vi "Configure Dialog.vi"(8 "error in (no error)":errorcluster, 11 "CAN Port Configuration in":T1={"CAN Interface"="CAN1", "XNET Cluster"="NIXNET_example.CAN_Cluster", "#Signals"=0, "Sample Rate (Hz)"=100.0} {"Sample Rate (Hz)" format="%#_13g"}) -> (0 "error out":errorcluster, 1 "Canceled?":bool, 3 "CAN Port Configuration out":T1={"CAN Interface"="CAN1", "XNET Cluster"="NIXNET_example.CAN_Cluster", "#Signals"=28, "Sample Rate (Hz)"=100.0} {"Sample Rate (Hz)" format="%#_13g"})   [LabVIEW 2021, in "XNET-CAN-Signal-Logger.lvlib"]
uses:
  XNET-CAN-Signal-Logger.lvlib
  Typedef/Def-CAN Port Configuration.ctl
  <resource>/objmgr/xnet.rc
panel:
  in  "Cancel":bool
  in  "OK":bool
  in  "CAN Port Configuration":T1={"CAN Interface"="CAN1", "XNET Cluster"="ManyXnetChannels", "#Signals"=0, "Sample Rate (Hz)"=100.0} {"Sample Rate (Hz)" format="%#_13g"}
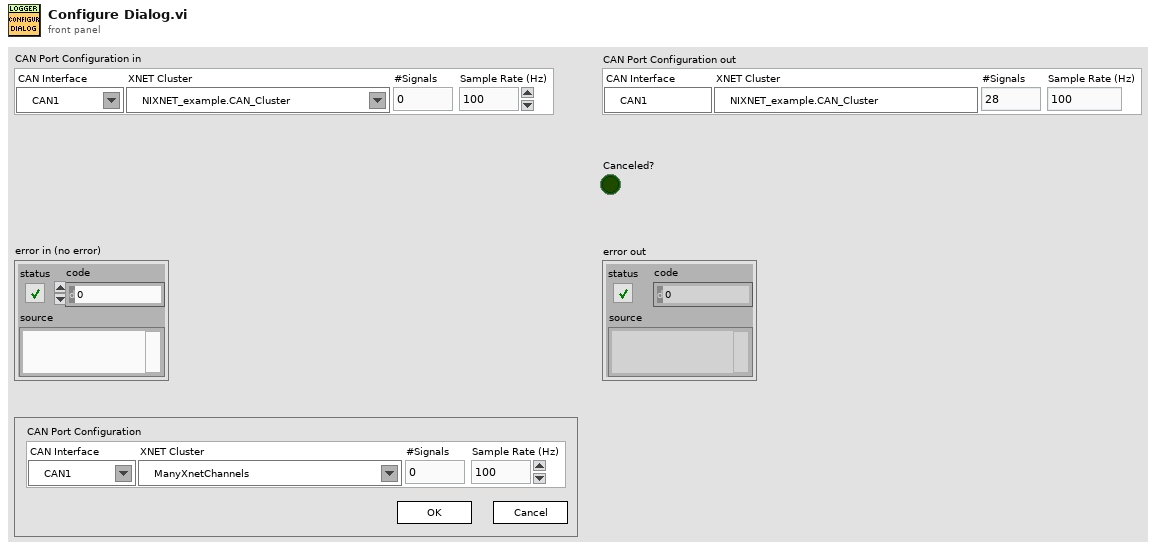
[diagram p1: front panel]
types:
  T1 = typedef "XNET-CAN-Signal-Logger.lvlib/Def-CAN Port Configuration.ctl" = cluster{"CAN Interface":refnum<k21>, "XNET Cluster":refnum<k21>, "#Signals":i32, "Sample Rate (Hz)":dbl}
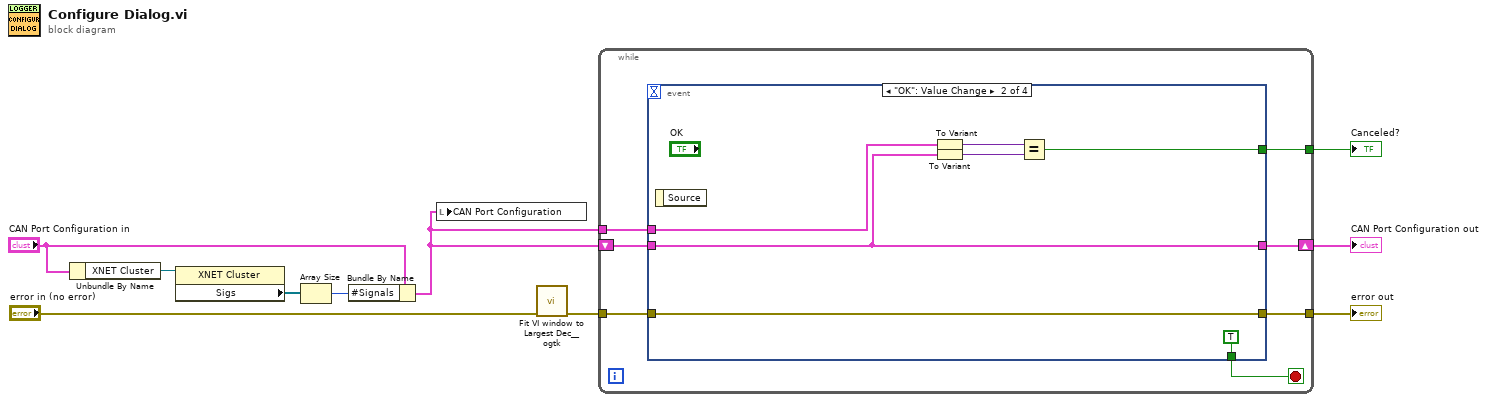
[diagram p0: block diagram]
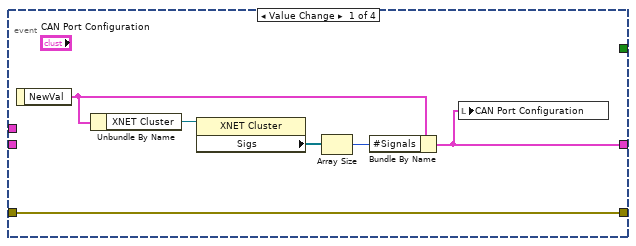
[diagram p2: hidden frame]
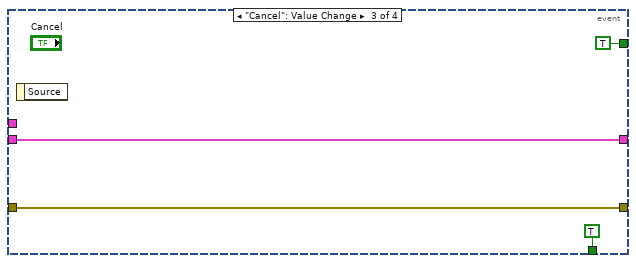
[diagram p3: hidden frame]
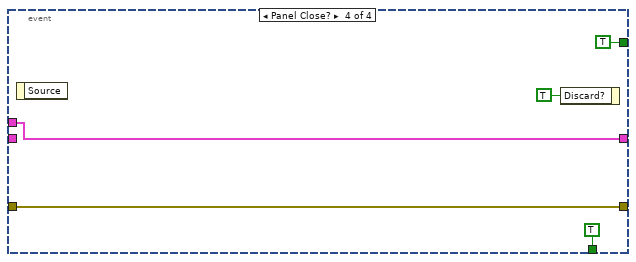
[diagram p4: hidden frame]
diagram:
  n1 = Unbundle By Name("CAN Port Configuration in") -> ("XNET Cluster"=w4:refnum<k21>)
  n2 = property class="XNET Cluster"(reference=w4) -> ("Sigs"=w6:refnum<k21>[])  [unwired: 1 in, 2 out]
  n3 = Array Size(array=w6) -> (size(s)=w5:i32)
  n4 = Bundle By Name(cluster="CAN Port Configuration in", "#Signals"=w5) -> (w2:T1)
  n5 = local write "CAN Port Configuration"(w2) -> ()
  n6 = call <userlib>:"Fit VI window to Largest Dec__ogtk.vi"("error in (no error)"="error in (no error)") -> ("error out"=w10:errorcluster)  [unwired: 5 in, 1 out]
  n7 = while {
    tunnel: w10 -> [w16]
    tunnel: [w17] -> w9
    tunnel: [w12] -> w7
    shift-right: [w14] -> w1
    shift-left: w2 -> [w13]
    tunnel: w2 -> [w11]
    stop <- w15 stop-if-true
    n8 = event shown="[1] \"OK\": Value Change" {
      selector: _ -> [_ _ _ _]
      dyn-events: _ -> [_ _ _ _]
      timeout: _ -> [_ _ _ _]
      tunnel: [w21 w30 w34 w39] -> w17
      tunnel: w16 -> [w21 w30 w34 w39]
      tunnel: [_ TRUE ("OK") TRUE ("OK") TRUE ("OK")] -> w15
      tunnel: [w18 w27 w32 w35] -> w14
      tunnel: w13 -> [_ w27 w32 _]
      tunnel: [_ w26 TRUE ("Cancel") TRUE ("Cancel")] -> w12
      tunnel: w11 -> [_ w28 _ w35]
      event Value Change {
        n9 = event-data() -> ("NewVal"=w19:T1)  [unwired: 1 in]
        n10 = Unbundle By Name(w19) -> ("XNET Cluster"=w20:refnum<k21>)
        n11 = property class="XNET Cluster"(reference=w20) -> ("Sigs"=w23:refnum<k21>[])  [unwired: 1 in, 2 out]
        n12 = Array Size(array=w23) -> (size(s)=w22:i32)
        n13 = Bundle By Name(cluster=w19, "#Signals"=w22) -> (w18:T1)
        n14 = local write "CAN Port Configuration"(w18) -> ()
      }
      event "OK": Value Change {
        n15 = event-data() -> ()  [unwired: 1 in, 1 out]
        n16 = To Variant(anything=w28) -> (Variant=w25:variant)
        n17 = To Variant(anything=w27) -> (Variant=w24:variant)
        n18 = Equal?(x=w25, y=w24) -> (x = y?=w26:bool)
      }
      event "Cancel": Value Change {
        n19 = event-data() -> ()  [unwired: 1 in, 1 out]
      }
      event Panel Close? {
        n20 = event-data() -> ()  [unwired: 1 in, 1 out]
        n21 = event-data("Discard?"=TRUE) -> ()  [unwired: 1 in, 1 out]
      }
    }
  }
  "error out" <- w9
  "CAN Port Configuration out" <- w1
  "Canceled?" <- w7
